vi "Copy CE template files for SS.vi"(7 "before SS? (T)":bool=TRUE, 8 "error in (no error)":errorcluster, 10 "CE template file":path, 11 "SS measurement":T1 {"PJVS reference voltages array of vector cluster"."PJVS reference voltages vector" format="%#_3p"; "PJVS frequencies (Hz)" format="%#_3p"; "Record lengths (multiples of periods)" format="%#_3p"; "Sampling frequencies (Hz)" format="%#_3p"; "Signal amplitudes (V)" format="%#_3p"; "Signal frequencies (Hz)" format="%#_3p"}) -> (0 "error out":errorcluster, 1 "new CE template FR fit mat file":path, 2 "new CE template file relative":path, 3 "new CE template file":path)   [LabVIEW 2020]
uses:
  SS Measurement/Type definitions/SS measurement.ctl
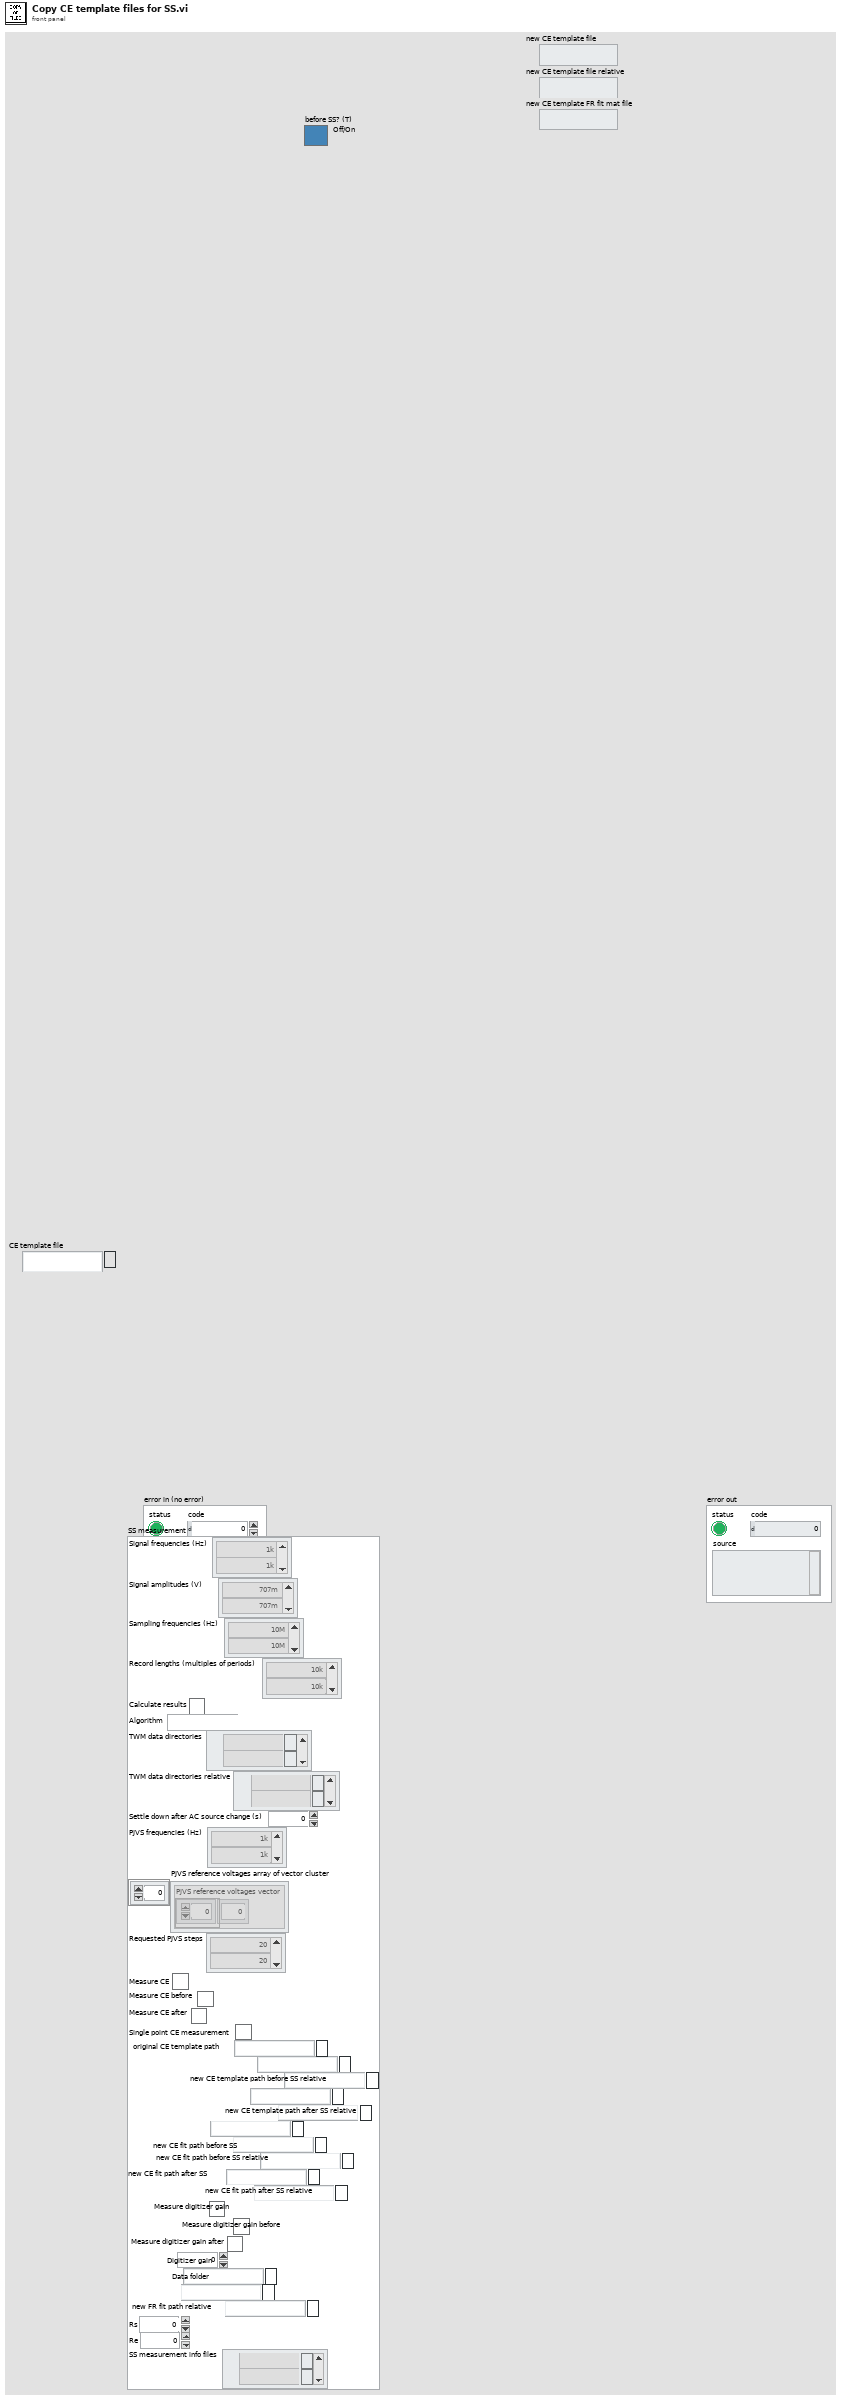
[diagram p1: front panel]
types:
  T1 = typedef "SS measurement.ctl" = cluster{"Signal frequencies (Hz)":dbl[], "Signal amplitudes (V)":dbl[], "Sampling frequencies (Hz)":dbl[], "Record lengths (multiples of periods)":dbl[], "Calculate results":bool, "Algorithm":string, "TWM data directories":path[], "TWM data directories relative":path[], "Settle down after AC source change (s)":dbl, "PJVS frequencies (Hz)":dbl[], "PJVS reference voltages array of vector cluster":cluster{"PJVS reference voltages vector":dbl[]}[], "Requested PJVS steps":u32[], "Measure CE":bool, "Measure CE before":bool, "Measure CE after":bool, "Single point CE measurement":bool, "original CE template path":path, "new CE template path before SS":path, "new CE template path before SS relative":path, "new CE template path after SS":path, "new CE template path after SS relative":path, "original CE fit path":path, "new CE fit path before SS":path, "new CE fit path before SS relative":path, "new CE fit path after SS":path, "new CE fit path after SS relative":path, "Measure digitizer gain":bool, "Measure digitizer gain before":bool, "Measure digitizer gain after":bool, "Digitizer gain":dbl, "Data folder":path, "FR fit path":path, "new FR fit path relative":path, "Rs":i32, "Re":i32, "SS measurement info files":path[]}
  T2 = typedef "Type definitions to be saved.ctl" = cluster{"Common properties":T3, "AC Source":T4, "DC meter":T6, "CE measurement":T8, "FR measurement":T9, "FR template":T10, "CE template":T11, "PJVS":T12, "SS measurement":T1, "AC sync source":T4}
  T3 = typedef "Common properties.ctl" = cluster{"Measurement status ref":refnum<vi>, "TWM Status ref":refnum<vi>, "Abort ref":refnum<vi>, "Skip waiting ref":refnum<vi>, "GNU Octave path":path, "TWM+QWTB path":path, "lvlib path":path, "TWM pipe":string, "PJVS status ref":refnum<vi>, "WAC path":path}
  T4 = typedef "AC Source.ctl" = cluster{"AC Source type":T5, "VISA":refnum<visa-resource-name>, "Ref. clock (Hz)":dbl, "status ref":refnum<vi>, "Fluke 57XX wideband output":bool, "Fluke 57XX ignore errors":bool, "Synchronization by AC signal":bool}
  T5 = typedef "AC Source type.ctl" = enum16{"Fluke 5XXX calibrator", "Tektronix AFG3000 series", "dummy", "Agilent 331xxA to 332xxA", "Agilent 335xxA to 336xxA"}
  T6 = typedef "DC meter.ctl" = cluster{"DC meter type":T7, "DC meter VISA":refnum<visa-resource-name>, "NPLC":dbl, "status ref":refnum<vi>}
  T7 = typedef "DC meter type.ctl" = enum16{"H/A/K 3458", "Fluke 8508A", "dummy", "Keithley 2182"}
  T8 = typedef "CE measurement.ctl" = cluster{"Signal frequencies (Hz) T":dbl[], "Signal amplitudes (V) T":dbl[], "Sampling frequencies (Hz) T":dbl[], "Record lengths (multiples of periods) T":dbl[], "TWM data root directory":path, "TWM mreasurements directories":path[], "Calculate RMS from samples":bool, "RMS algorithm T":string, "Settle down after AC source change (s) T":dbl, "Skip PJVS setup":bool, "Measurement template file":path, "Row of START keyword T":i32, "Row of STOP keyword T":i32, "Measurement template line T":i32[], "Switch position T":dbl[], "FR fit mat file T":path, "Recalculate-skip already calculated":bool}
  T9 = typedef "FR measuement.ctl" = cluster{"Measurement frequencies (Hz)":dbl[], "Sampling frequency (Hz)":dbl, "Signal amplitude (V)":dbl, "AC-DC settle time (s)":dbl, "Record length (multiples of period)":dbl[], "Measurement template file":path, "Row of START keyword":i32, "Row of STOP keyword":i32, "Calculate RMS from samples":bool, "AC-DC warm up time (s)":dbl, "Measurement template line":i32[], "DC meter readings No.":i32, "Algorithm":string, "Simultaneous measurement":bool, "Recalculate-skip already calculated":bool}
  T10 = typedef "FR template.ctl" = cluster{"Keywords column":i32, "Sig. freq. column":i32, "Rec. len. column":i32, "Meas. points. row min to read":i32, "Meas. points. row max to read":i32, "Properties column":i32, "Properties row start":i32, "Properties row end":i32, "Keyword START regexp":string, "Keyword STOP regexp":string, "HW data column":i32, "HW data row start":i32, "HW data row end":i32, "TIme and date column start":i32, "Digitizer value column start ":i32, "DC mean column start ":i32, "DC readings column start":i32}
  T11 = typedef "CE template.ctl" = cluster{"Keywords column":i32, "Sig. freq. column":i32, "Rec. len. column":i32, "Switch pos column":i32, "Meas. points. row min to read":i32, "Meas. points. row max to read":i32, "Properties column":i32, "Properties row start":i32, "Properties row end":i32, "Keyword START regexp":string, "Keyword STOP regexp":string, "HW data column":i32, "HW data row start":i32, "HW data row end":i32, "TIme and date column start":i32, "Digitizer value column start ":i32}
  T12 = typedef "PJVS.ctl" = cluster{"PJVS type":T13, "Status Refnum":refnum<vi>, "AC-supraVOLTcontrol":cluster{"IP address:port (0.0.0.0:0000)":string, "Timeouts":T14, "Simulation mode":bool, "Debug mode":bool}, "NPL bias source":cluster{"DataSocketCluster":T15}, "Manual PJVS":cluster{"PJVS frequency (Hz)":dbl, "Reference voltages (V)":dbl[], "File with PJVS voltages":path}, "VTT PJVS":cluster{"some VTT only property":string}}
  T13 = typedef "PJVS Type.ctl" = enum16{"AC-supraVOLTcontrol", "JV modified NPL bias control", "Manual PJVS", "VTT PJVS"}
  T14 = typedef "ACSVcontrol-driver.lvlib/Timeouts.ctl" = cluster{"TCP Read & Write (ms)":i32, "Sensors readout":i32, "PJVS setup":i32, "Nullmeter readout":i32, "Multiplexer setup":i32, "57XX setup":i32, "Generator setup":i32, "Synthesizer setup":i32, "Sampler readout":i32}
  T15 = typedef "DataSocketCluster external.ctl" = cluster{"Server Machine":string, "Client Machine":string, "Data":string, "TimeStamp":dbl, "Count":i32, "Target Process":string}
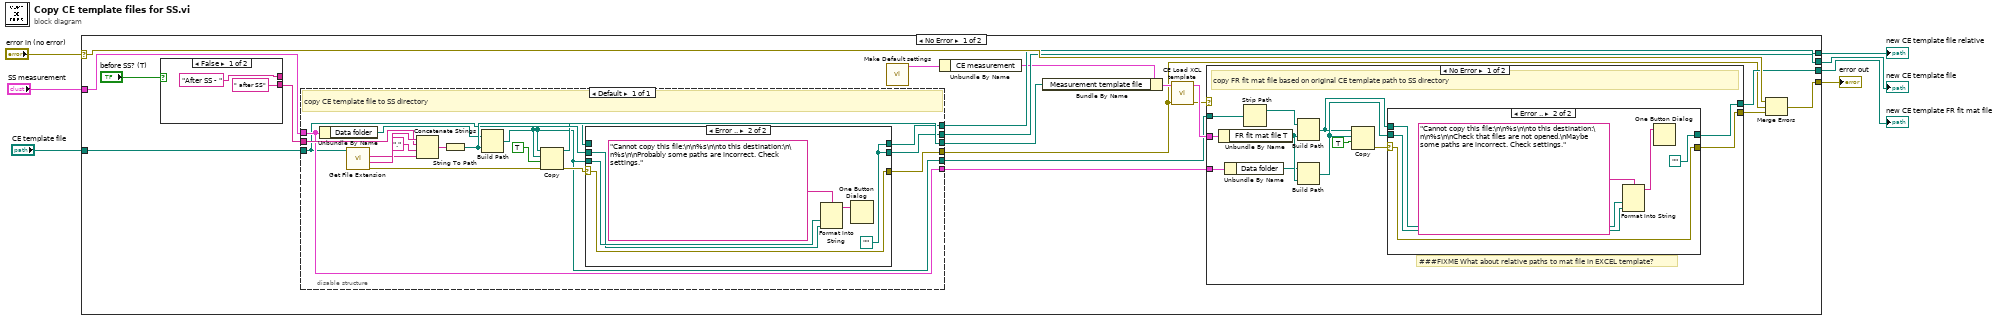
[diagram p0: block diagram]
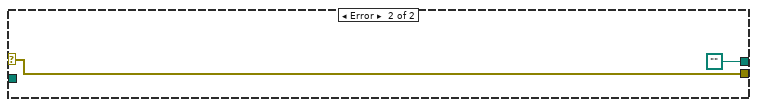
[diagram p3: hidden frame]
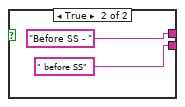
[diagram p5: hidden frame]
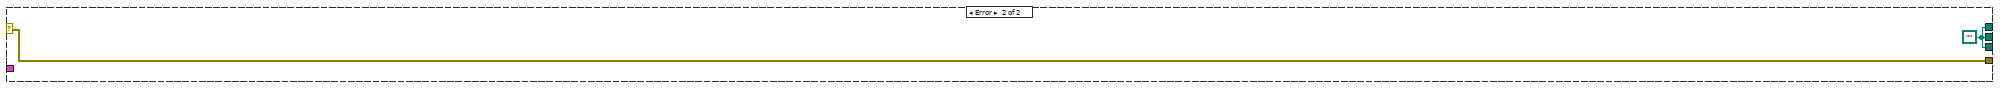
[diagram p6: hidden frame]
diagram:
  n1 = case shown="No Error" "error in (no error)" {
    selector: "error in (no error)" -> [w23 w80]
    tunnel: [w26 w80] -> w7
    tunnel: [w20 w79] -> w5
    tunnel: [w19 w79] -> w4
    tunnel: [w18 w79] -> w3
    tunnel: "SS measurement" -> [w12 _]
    tunnel: "CE template file" -> [w8 _]
    frame No Error {
      n2 = case shown="False" "before SS? (T)" {
        tunnel: ["After SS - " ("name suffix ()") "Before SS - " ("name suffix ()")] -> _
        tunnel: [" after SS" ("string") " before SS" ("string")] -> w24
        frame False {
        }
        frame True {
        }
      }
      n3 = disable-structure shown="Default" {
        disable-tunnel: w24 -> [w62]
        disable-tunnel: [w57] -> w13
        disable-tunnel: [w55] -> w22
        disable-tunnel: [w54] -> w20
        disable-tunnel: [w53] -> w19
        disable-tunnel: [w49] -> w15
        disable-tunnel: w12 -> [w50]
        disable-tunnel: [w50] -> w11
        disable-tunnel: w8 -> [w49]
        frame Enabled {
          # "copy CE template file to SS directory"
          n4 = Unbundle By Name(w50) -> ("Data folder"=w51:path)
          n5 = call <vilib>:"Get File Extension.vi"("file"=w49) -> ("error out"=w59:errorcluster, "filename without extension"=w63:string, "lowercase file extension"=w60:string)  [unwired: 6 in, 2 out]
          n6 = Concatenate Strings(w63, w62, "." ("string"), w60) -> (w64:string)
          n7 = String To Path(string=w64) -> (path=w52:path)
          n8 = Build Path(base path=w51, name or relative path=w52) -> (appended path=w56:path)
          n9 = Copy(8:w59, 9:TRUE ("overwrite (F)"), 10:w56, 11:w49) -> (0:w58:errorcluster, 3:w55:path)  [unwired: 1 in, 1 out]
          n10 = case shown="Error .." w58 {
            selector: w58 -> [w68 w72]
            tunnel: [w68 w72] -> w57
            tunnel: w49 -> [_ w71]
            tunnel: w56 -> [w67 w70]
            tunnel: [w67 w69] -> w54
            tunnel: [w66 w69] -> w53
            tunnel: w52 -> [w66 _]
            frame No Error {
            }
            frame Error {
              w69 = path ""
              n11 = Format Into String(format string="Cannot copy this file:\n\n%s\n\nto this destination:\n\n%s\n\nProbably some paths are incorrect. Check settings.", w71, w70) -> (resulting string=w73:string)  [unwired: 2 in, 1 out]
              n12 = One Button Dialog(message=w73) -> ()  [unwired: 1 in, 1 out]
            }
          }
        }
      }
      n13 = call "Make Default settings.vi"() -> ("TD to be saved"=w10:T2)  [unwired: 11 in]
      n14 = Unbundle By Name(w10) -> ("CE measurement"=w9:T8)
      n15 = Bundle By Name(cluster=w9, "Measurement template file"=w22) -> (w17:T8)
      n16 = call "CE Load XCL template.vi"("error in (no error)"=w13, "CE measurement"=w17) -> ("error out"=w14:errorcluster, "CE measurement out"=w16:T8)  [unwired: 8 in]
      n17 = case shown="No Error" w14 {
        selector: w14 -> [_ w48]
        tunnel: [w38 w48] -> w21
        tunnel: [w37 path ""] -> w18
        tunnel: w16 -> [w36 _]
        tunnel: w15 -> [w35 _]
        tunnel: w11 -> [w28 _]
        frame No Error {
          # "###FIXME What about relative paths to mat file in EXCEL template?"
          # "copy FR fit mat file based on original CE template path to SS directory"
          n18 = Unbundle By Name(w36) -> ("FR fit mat file T"=w32:path)
          n19 = Unbundle By Name(w28) -> ("Data folder"=w27:path)
          n20 = Strip Path(path=w35) -> (stripped path=w29:path)  [unwired: 1 out]
          n21 = Build Path(base path=w29, name or relative path=w32) -> (appended path=w30:path)
          n22 = Build Path(base path=w27, name or relative path=w32) -> (appended path=w31:path)
          n23 = Copy(9:TRUE ("overwrite (F)"), 10:w31, 11:w30) -> (0:w33:errorcluster)  [unwired: 2 in, 2 out]
          n24 = case shown="Error .." w33 {
            selector: w33 -> [w40 w44]
            tunnel: [w40 w44] -> w38
            tunnel: w30 -> [_ w43]
            tunnel: w31 -> [w39 w42]
            tunnel: [w39 path ""] -> w37
            frame No Error {
            }
            frame Error {
              n25 = Format Into String(format string="Cannot copy this file:\n\n%s\n\nto this destination:\n\n%s\n\nCheck that files are not opened.\nMaybe some paths are incorrect. Check settings.", w43, w42) -> (resulting string=w45:string)  [unwired: 2 in, 1 out]
              n26 = One Button Dialog(message=w45) -> ()  [unwired: 1 in, 1 out]
            }
          }
        }
        frame Error {
        }
      }
      n27 = Merge Errors(w23, w13, w21) -> (w26:errorcluster)
    }
    frame Error {
      w79 = path ""
    }
  }
  "error out" <- w7
  "new CE template file" <- w5
  "new CE template file relative" <- w4
  "new CE template FR fit mat file" <- w3
